vi "TestLocalizeLooped.vi"() -> ()   [LabVIEW 2011]
uses:
  TrackerDLL.vi
panel:
  out "X profile":sgl[](graph)
  out "Y profile":sgl[](graph)
  out "Y result":sgl[](graph)
  out "True Y":dbl
  out "True X":dbl
  out "COM results":cluster{dbl, dbl}(graph)
  out "XCor results":cluster{dbl, dbl}(graph)
  in  "y center":dbl=128.0
  in  "x center":dbl=128.0 min=40.0 max=200.0
  out "X result":sgl[](graph)
  in  "spotsize":sgl(knob)=20.0 min=1 max=20 scale=0.0..10.0
  in  "Boolean":bool
  out "debug":T1(plugin-control)
  out "median":sgl
  out "xcorpos":cluster{"XCor X":sgl, "XCor Y":sgl}
  out "COM":cluster{"comX":sgl, "comY":sgl}
  out "Image":T1(plugin-control)
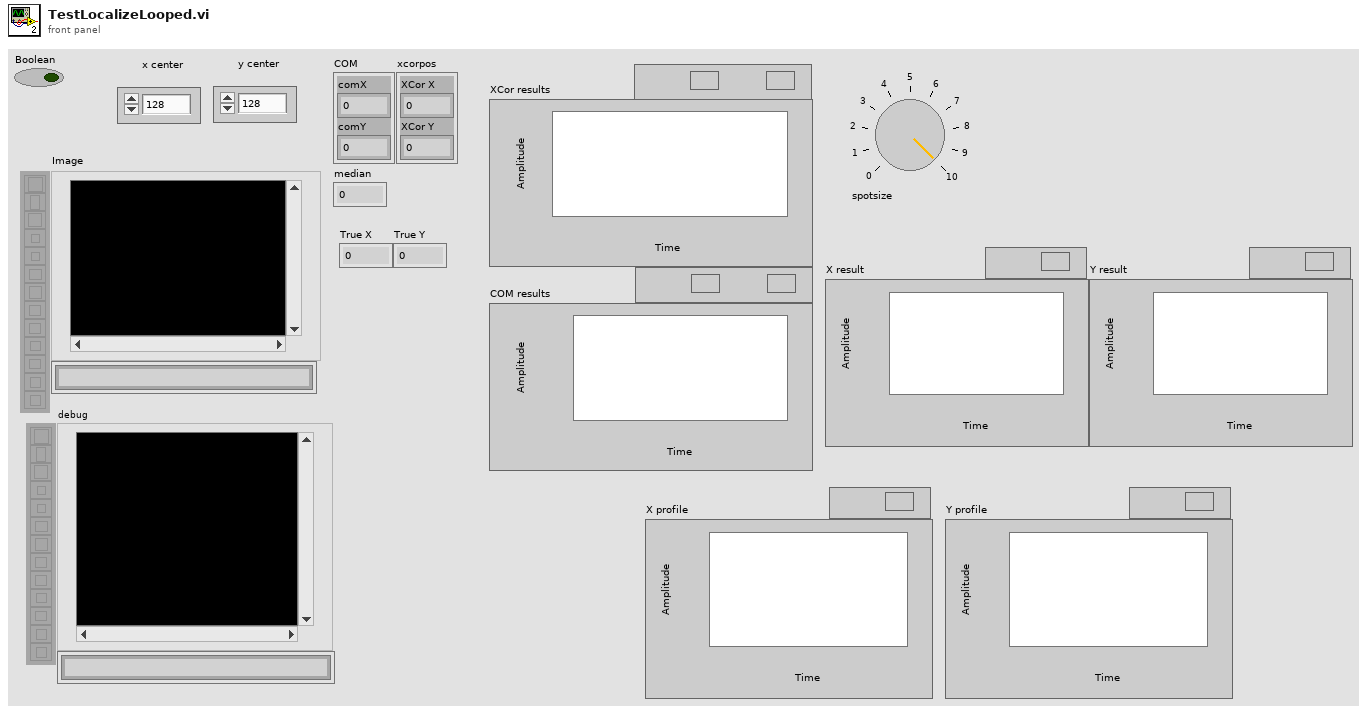
[diagram p1: front panel]
types:
  T1 = typedef "IMAQ Image.ctl" = refnum<image>
  T2 = typedef "Image Type" = u32
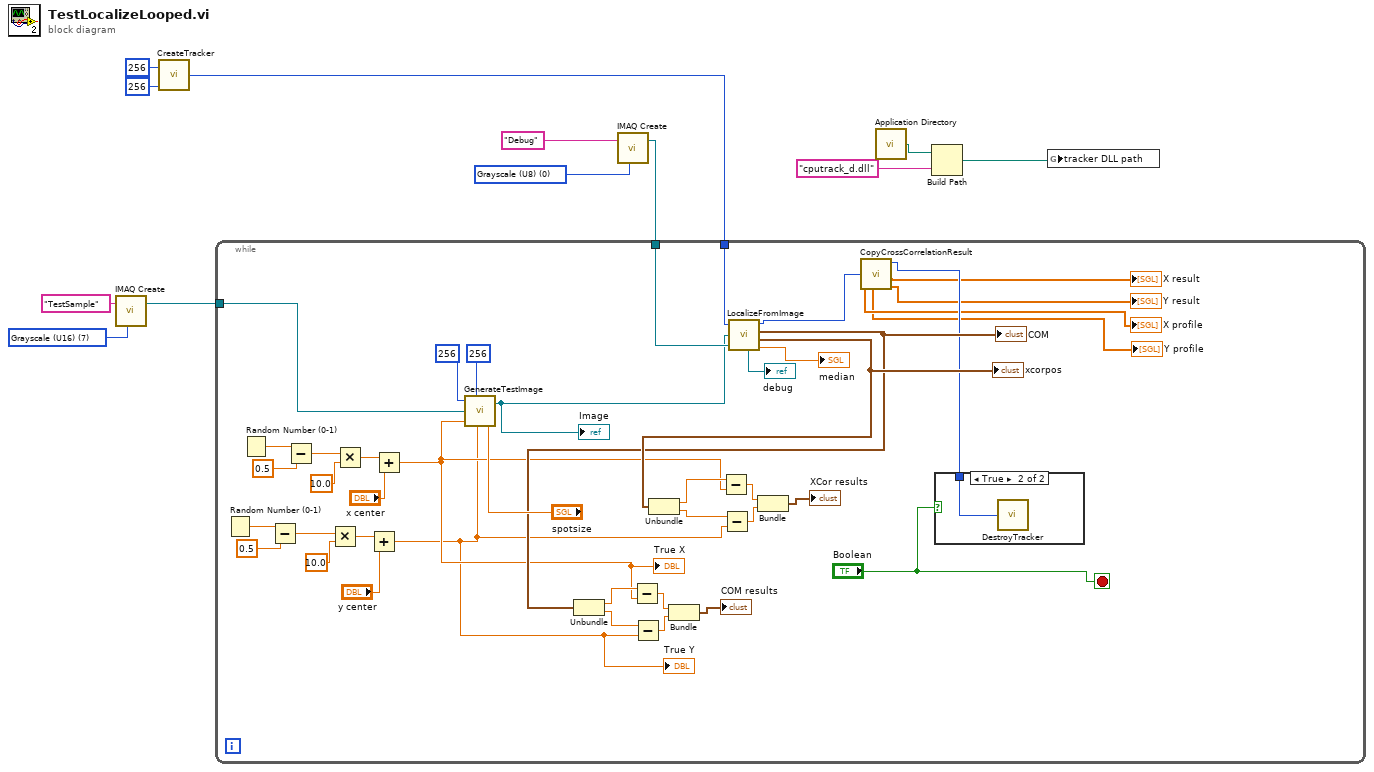
[diagram p0: block diagram]
diagram:
  w2 = T2 7 items=["Grayscale (U8)", "Grayscale (I16)", "Grayscale (SGL)", "Complex (CSG)", "RGB (U32)", "HSL (U32)", "RGB (U64)", "Grayscale (U16)"] ("Image Type")
  w11 = T2 0 items=["Grayscale (U8)", "Grayscale (I16)", "Grayscale (SGL)", "Complex (CSG)", "RGB (U32)", "HSL (U32)", "RGB (U64)", "Grayscale (U16)"] ("Image Type")
  n1 = call "IMAQ Create"("Image Name"="TestSample" ("String"), "Image Type"=w2) -> ("New Image"=w1:T1)  [unwired: 3 in, 1 out]
  n2 = call "CreateTracker.vi"("height"=u32 256, "width"=u32 256) -> ("return type"=w4:u64)
  n3 = call "IMAQ Create"("Image Name"="Debug" ("String"), "Image Type"=w11) -> ("New Image"=w5:T1)  [unwired: 3 in, 1 out]
  n4 = while {
    tunnel: w5 -> [w54]
    tunnel: w4 -> [w53]
    tunnel: w1 -> [w48]
    stop <- "Boolean" stop-if-true
    n5 = Random Number (0-1)() -> (number: 0 to 1=w35:dbl)
    n6 = Random Number (0-1)() -> (number: 0 to 1=w39:dbl)
    n7 = Subtract(x=w35, y=0.5) -> (x-y=w33:dbl)
    n8 = Subtract(x=w39, y=0.5) -> (x-y=w36:dbl)
    n9 = Multiply(x=w33, y=sgl 10.0) -> (x*y=w42:dbl)
    n10 = Multiply(x=w36, y=sgl 10.0) -> (x*y=w44:dbl)
    n11 = Add(x=w42, y="y center") -> (x+y=w19:dbl)
    "True Y" <- w19
    n12 = Add(x=w44, y="x center") -> (x+y=w20:dbl)
    "True X" <- w20
    n13 = call "GenerateTestImage.vi"("width"=u32 256, "height"=u32 256, "image"=w48, "xpos"=w20, "ypos"=w19, "spotsize"="spotsize") -> ("Image"=w46:T1)
    "Image" <- w46
    n14 = call "LocalizeFromImage.vi"("tracker"=w53, "input image"=w46, "debug image"=w54) -> ("tracker"=w18:u64, "COM"=w23:cluster{"comX":sgl, "comY":sgl}, "debug image"=→"debug":T1, "xcorpos"=w32:cluster{"XCor X":sgl, "XCor Y":sgl}, "median"=→"median":sgl)  [unwired: 3 in]
    "COM" <- w23
    "xcorpos" <- w32
    n15 = Unbundle(w23) -> ("comX"=w22:sgl, "comY"=w21:sgl)
    n16 = Subtract(x=w22, y=w20) -> (x-y=w26:dbl)
    n17 = Subtract(x=w21, y=w19) -> (x-y=w25:dbl)
    n18 = Unbundle(w32) -> ("XCor X"=w31:sgl, "XCor Y"=w30:sgl)
    n19 = Bundle(w26, w25) -> (→"COM results":cluster{dbl, dbl})  [unwired: 1 in]
    n20 = Subtract(x=w31, y=w20) -> (x-y=w29:dbl)
    n21 = Subtract(x=w30, y=w19) -> (x-y=w28:dbl)
    n22 = Bundle(w29, w28) -> (→"XCor results":cluster{dbl, dbl})  [unwired: 1 in]
    n23 = call "CopyCrossCorrelationResult.vi"("tracker"=w18) -> ("x prof"=→"X profile":sgl[], "y prof"=→"Y profile":sgl[], "tracker"=w17:u64, "x result"=→"X result":sgl[], "y_result"=→"Y result":sgl[])  [unwired: 3 in]
    n24 = case shown="True" "Boolean" {
      tunnel: w17 -> [_ w55]
      frame False {
      }
      frame True {
        n25 = call "DestroyTracker.vi"("tracker"=w55) -> ()
      }
    }
  }
  n26 = call <vilib>:"Application Directory.vi"() -> ("Application Directory"=w10:path)
  n27 = Build Path(base path=w10, name or relative path="cputrack_d.dll") -> (appended path=w8:path)
  n28 = global write "TrackerDLL.vi" "tracker DLL path"(w8) -> ()
